vi "ex4_good.vi"() -> ()   [LabVIEW 2022 SP3]
uses:
  baa26b7c-edc6-4099-a58f-b2071b499866.vi
  <vilib>/Array/Sort 2D Array - Pop Stack.vi
  <vilib>/Array/Sort 2D Array - Push Stack.vi
panel:
  in  "Age":i32
  in  "Nationality":string
  in  "Surname":string
  in  "Name":string
  out "User List":string
  in  "Enum":T1(ring)
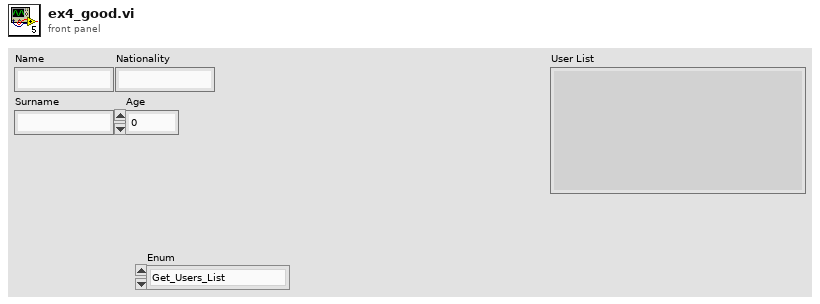
[diagram p1: front panel]
types:
  T1 = enum16{"Get_Users_List", "Add_User", "Clear_User_List"}
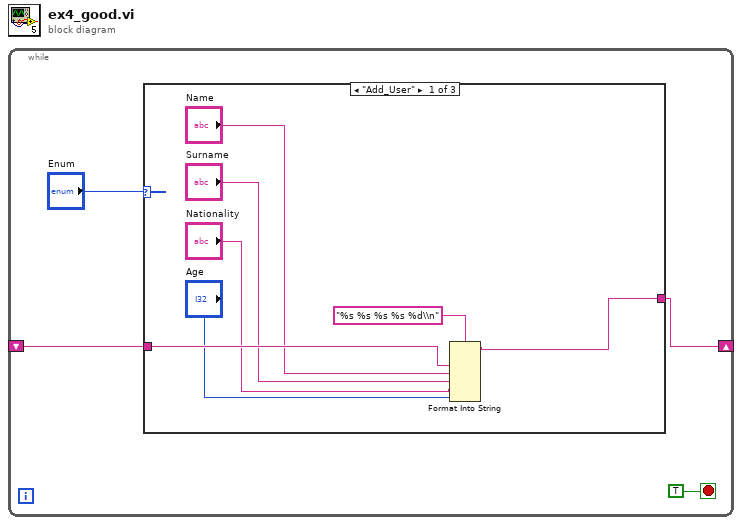
[diagram p0: block diagram]
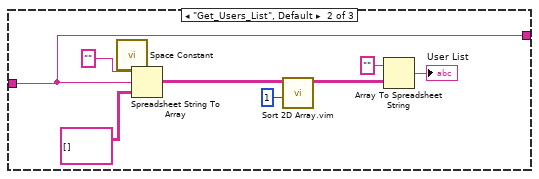
[diagram p2: hidden frame]
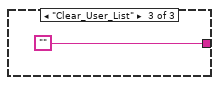
[diagram p3: hidden frame]
diagram:
  n1 = while {
    shift-right: [w1] -> _
    shift-left: _ -> [w2]
    stop <- TRUE stop-if-true
    n2 = case shown="\"Add_User\"" "Enum" {
      tunnel: w2 -> [w9 w17 _]
      tunnel: [w10 w17 ""] -> w1
      frame "Add_User" {
        n3 = Format Into String(format string="%s %s %s %s %d\\n", w9, "Name", "Surname", "Nationality", "Age") -> (resulting string=w10:string)  [unwired: 2 in, 1 out]
      }
      frame "Get_Users_List", Default {
        n4 = call <vilib>:"Space Constant.vi"() -> ("String"=w19:string)
        n5 = Spreadsheet String To Array(delimiter (Tab)=w19, format string="", spreadsheet string=w17, array type (2D Dbl)=string[][] []) -> (array=w15:string[][])
        n6 = call "Sort 2D Array.vim"("index"=1, "2D array"=w15) -> ("sorted 2D array"=w14:string[][])  [unwired: 8 in, 1 out]
        n7 = Array To Spreadsheet String(array=w14, 3:"" ("format string")) -> (spreadsheet string=→"User List":string)  [unwired: 1 in]
      }
      frame "Clear_User_List" {
      }
    }
  }
